vi "iRobot Drive Direction.vi"(8 "error in":errorcluster, 9 "Velocity (mm/s)":i16, 10 "iRobot Drive Direction":T1, 11 "UART port in":T2) -> (0 "error out":errorcluster, 3 "UART port out":T2)   [LabVIEW 2010]
doc: "Drive the robot straight, clockwise, or counter-clockwise.\n\nThis VI writes to, but does not read from, the serial port."
uses:
  UART/UART Port Type.ctl
  Actuator Controls/iRobot Drive Direction.ctl
  Open Interface Controls/iRobot OpCode.ctl
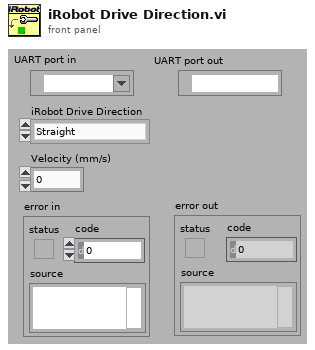
[diagram p1: front panel]
types:
  T1 = typedef "iRobot Drive Direction.ctl" = enum16{"Straight", "Clockwise", "Counter-Clockwise"}
  T2 = typedef "UART Port Type.ctl" = refnum<visa-resource-name>
  T3 = typedef "iRobot OpCode.ctl" = u8
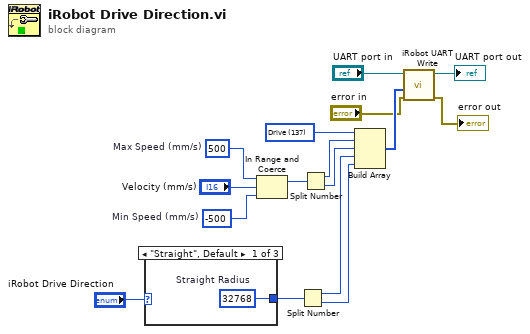
[diagram p0: block diagram]
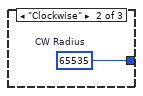
[diagram p2: hidden frame]
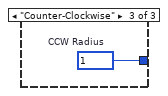
[diagram p3: hidden frame]
diagram:
  w14 = i16 -500  # Min Speed (mm/s)
  w15 = i16 500  # Max Speed (mm/s)
  w8 = T3 137 items=["Start"=128, "Baud"=129, "Control"=130, "Safe"=131, "Full"=132, "Demo"=136, "Demo - Cover"=135, "Demo - Cover and Dock"=143, "Demo - Spot"=134, "Drive"=137, "Drive Direct"=145, "LEDs"=139, "Digital Outputs"=147, "PWM Low Side Drivers"=144, "Low Side Drivers"=138, "Send IR"=151, "Song"=140, "Play Song"=141, "Sensors"=142, "Query List"=149, "Stream"=148, "Pause/Resume Stream"=150, "Script"=152, "Play Script"=153, "Show Script"=154, "Wait Time"=155, "Wait Distance"=156, "Wait Angle"=157, "Wait Event"=158] ("OpCode")
  n1 = case shown="\"Straight\", Default" "iRobot Drive Direction" {
    tunnel: [w17 w18 w19] -> w1
    frame "Straight", Default {
      w17 = u16 32768  # Straight Radius
    }
    frame "Clockwise" {
      w18 = u16 65535  # CW Radius
    }
    frame "Counter-Clockwise" {
      w19 = u16 1  # CCW Radius
    }
  }
  n2 = In Range and Coerce(upper limit=w15, x="Velocity (mm/s)", lower limit=w14) -> (coerced(x)=w13:i16)  [unwired: 1 out]
  n3 = Split Number(x=w1) -> (hi(x)=w10:u8, lo(x)=w9:u8)
  n4 = Split Number(x=w13) -> (hi(x)=w12:u8, lo(x)=w11:u8)
  n5 = Build Array(w8, w12, w11, w10, w9) -> (w7:T3[])
  n6 = call "iRobot UART Write.vi"("error in"="error in", "data"=w7, "UART port in"="UART port in") -> ("error out"=→"error out":errorcluster, "UART port out"=→"UART port out":T2)  [unwired: 7 in]
